vi "issue_init_with_peers_response.vi"(5 "error in (no error)":errorcluster) -> (19 "error out":errorcluster)   [LabVIEW 2016]
uses:
  support/controls/queue_assistant_actions.ctl
  support/controls/entity.ctl
  support/controls/entity_type.ctl
  support/controls/response.ctl
  support/controls/response_type.ctl
  support/controls/queue_type.ctl
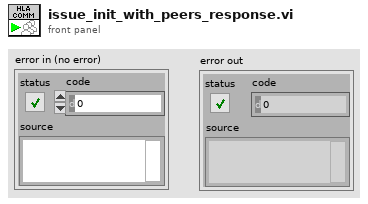
[diagram p1: front panel]
types:
  T1 = typedef "entity.ctl" = cluster{"type":T2, "classPath":string, "params":string[][], "instanceName":string}
  T2 = typedef "entity_type.ctl" = string
  T3 = typedef "queue_assistant_actions.ctl" = enum16{"--- unused ---", "bulk_enq_ahead", "bulk_enq_behind", "destroy", "empty?", "enq_ahead", "enq_behind", "flush", "get_queues", "init"}
  T4 = typedef "queue_type.ctl" = enum16{"all", "dostep", "entities_incoming", "entities_outoing", "response"}
  T5 = typedef "response_type.ctl" = string
  T6 = typedef "response.ctl" = cluster{"respType":T5, "flattenedContent":string}
  T7 = typedef "queue_references.ctl" = cluster{"entities_in":refnum<queue>, "entities_out":refnum<queue>, "timestep":refnum<queue>, "response":refnum<queue>}
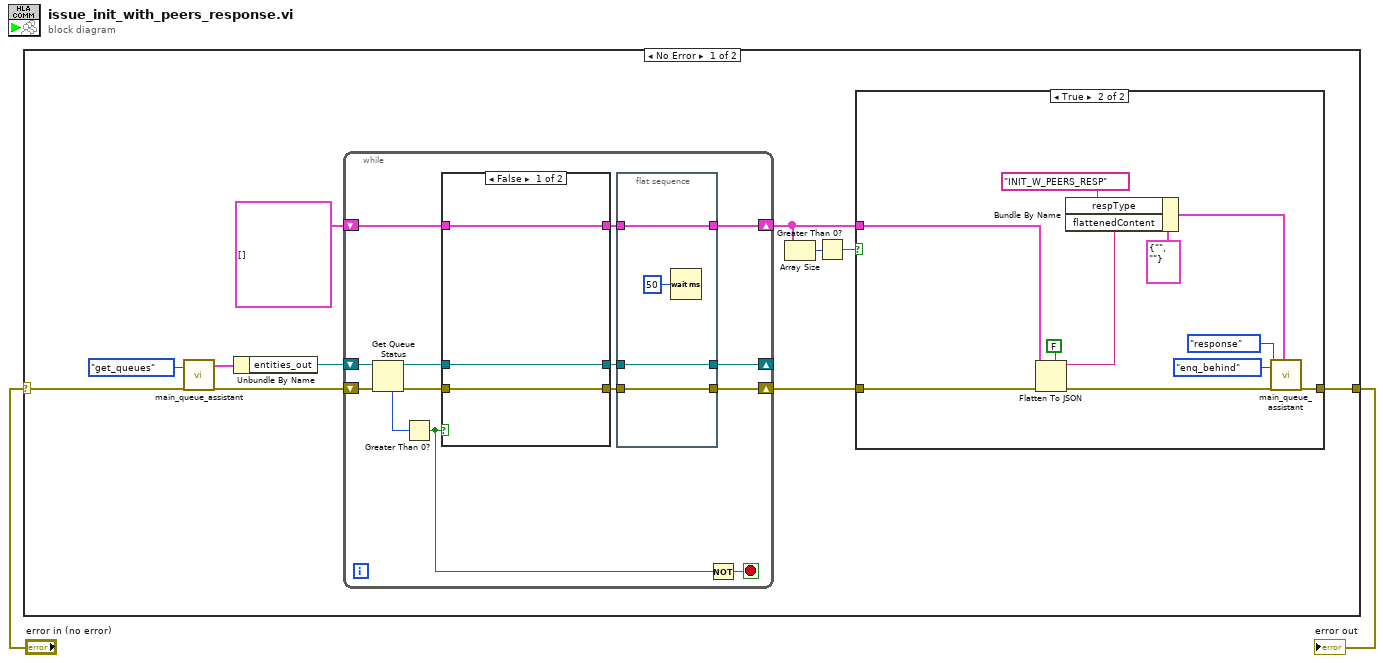
[diagram p0: block diagram]
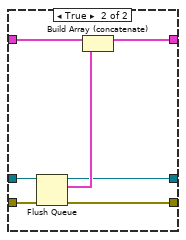
[diagram p3: hidden frame]
diagram:
  n1 = case shown="No Error" "error in (no error)" {
    selector: "error in (no error)" -> [w4 w54]
    tunnel: [w3 w54] -> w1
    frame No Error {
      n2 = call "main_queue_assistant.vi"("action (enq_behind = def)"=queue_assistant_actions."get_queues", "error in (no error)"=w4) -> ("refs (out)"=w12:T7, "error out"=w10:errorcluster)  [unwired: 15 in, 1 out]
      n3 = Unbundle By Name(w12) -> ("entities_out"=w11:refnum<queue>)
      n4 = while {
        shift-right: [w28] -> w7
        shift-left: T1[] [] ("remaining elements") -> [w34]
        shift-right: [w27] -> _
        shift-left: w11 -> [w39]
        shift-right: [w26] -> w8
        shift-left: w10 -> [w38]
        stop <- w32 stop-if-true
        n5 = Get Queue Status(queue=w39, error in (no error)=w38) -> (queue out=w36:refnum<queue>, error out=w35:errorcluster, # elements in queue=w37:i32)  [unwired: 1 in, 5 out]
        n6 = Greater Than 0?(x=w37) -> (x > 0?=w33:bool)
        n7 = case shown="False" w33 {
          tunnel: w36 -> [w45 w53]
          tunnel: w35 -> [w44 w52]
          tunnel: w34 -> [w46 w51]
          tunnel: [w45 w49] -> w30
          tunnel: [w44 w48] -> w29
          tunnel: [w46 w47] -> w31
          frame False {
          }
          frame True {
            n8 = Flush Queue(queue=w53, error in (no error)=w52) -> (queue out=w49:refnum<queue>, remaining elements=w50:T1[], error out=w48:errorcluster)
            n9 = Build Array (concatenate)(w51, w50) -> (w47:T1[])
          }
        }
        n10 = flat-sequence {
          tunnel: [w43] -> w28
          tunnel: w31 -> [w43]
          tunnel: [w42] -> w27
          tunnel: w30 -> [w42]
          tunnel: [w41] -> w26
          tunnel: w29 -> [w41]
          frame #0 {
            n11 = Wait (ms)(milliseconds to wait=u32 50) -> ()  [unwired: 1 out]
          }
        }
        n12 = Not(x=w33) -> (.not. x?=w32:bool)
      }
      n13 = Array Size(array=w7) -> (size(s)=w6:i32)
      n14 = Greater Than 0?(x=w6) -> (x > 0?=w5:bool)
      n15 = case shown="True" w5 {
        tunnel: w8 -> [w14 w24]
        tunnel: w7 -> [_ w15]
        tunnel: [w14 w16] -> w3
        frame False {
        }
        frame True {
          n16 = Flatten To JSON(enable LabVIEW extensions? (T)=FALSE, anything=w15, error in (no error)=w24) -> (JSON string=w22:string, 11:w18:errorcluster)
          n17 = Bundle By Name(cluster=T6 {"respType"="", "flattenedContent"=""} ("response"), "respType"=T5 "INIT_W_PEERS_RESP", "flattenedContent"=w22) -> (w17:T6)
          n18 = call "main_queue_assistant.vi"("queue_type (def=all)"=queue_type."response", "action (enq_behind = def)"=queue_assistant_actions."enq_behind", "error in (no error)"=w18, "response"=w17) -> ("error out"=w16:errorcluster)  [unwired: 13 in, 2 out]
        }
      }
    }
    frame Error {
    }
  }
  "error out" <- w1
